vi "Render.vi"(7 "Renderer":refnum<class "Renderer.lvclass">, 8 "error in (no error)":errorcluster, 9 "Position":refnum<class "Vector 2D.lvclass">, 10 "String":string, 11 "Font in":refnum<class "Sprite Font.lvclass">) -> (0 "error out":errorcluster)   [LabVIEW 2021, in "Sprite Font.lvclass"]
uses:
  Sprite Font.lvclass
  Renderer/Renderer.lvclass
  Re-use Libraries/Vector 2D/Vector 2D.lvclass
  Sprite Font.lvclass/Sprite Font.ctl
  Re-use Libraries/Vector 2D/Vector 2D.lvclass/Vector 2D.ctl
  Renderer/Renderer.lvclass/Renderer.ctl
  Texture/Texture.lvclass/Texture.ctl
  Resource Manager/Resource Manager.lvclass
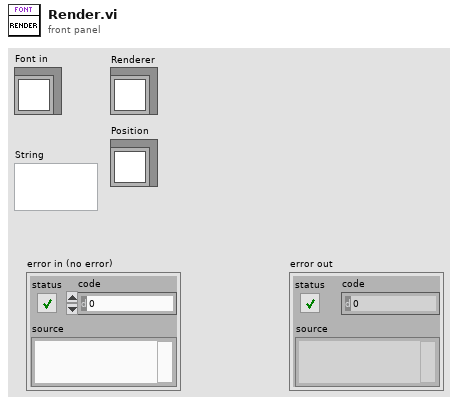
[diagram p1: front panel]
types:
  T1 = typedef "Sprite Font.lvclass/Character.ctl" = cluster{"Texture Name":string, "Size":refnum<class "Vector 2D.lvclass">}
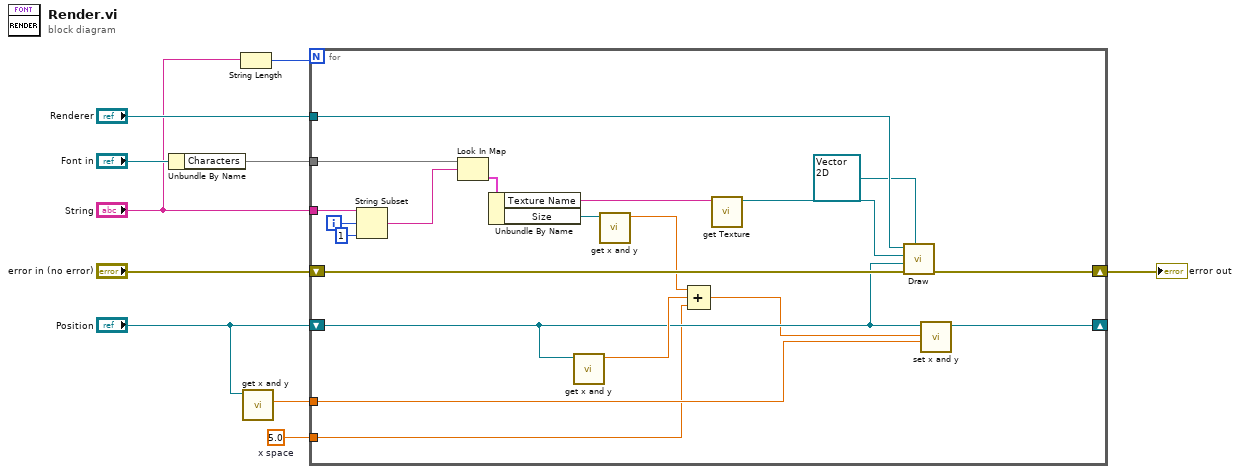
[diagram p0: block diagram]
diagram:
  w3 = sgl 5.0  # x space
  n1 = Unbundle By Name("Font in") -> ("Characters"=w6:map{string, T1})
  n2 = String Length(string="String") -> (length=w5:i32)
  n3 = call "get x and y.vi"("Vector 2D in"="Position") -> ("y"=w1:sgl)  [unwired: 9 in, 1 out]
  n4 = for {
    N: w5 -> [_]
    tunnel: "Renderer" -> [w30]
    shift-right: [w28] -> w9
    shift-left: "error in (no error)" -> [w27]
    tunnel: w6 -> [w18]
    shift-right: [w21] -> _
    shift-left: "Position" -> [w20]
    tunnel: w1 -> [w23]
    tunnel: "String" -> [w17]
    tunnel: w3 -> [w12]
    i -> [w16]
    n5 = String Subset(string=w17, offset (0)=w16, length (rest)=1 ("length (rest)")) -> (substring=w13:string)
    n6 = Look In Map(map=w18, key=w13) -> (value=w14:T1)  [unwired: 1 in, 1 out]
    n7 = Unbundle By Name(w14) -> ("Texture Name"=w25:string, "Size"=w24:refnum<class "Vector 2D.lvclass">)
    n8 = call "get x and y.vi"("Vector 2D in"=w20) -> ("x"=w22:sgl)  [unwired: 9 in, 1 out]
    n9 = call "get x and y.vi"("Vector 2D in"=w24) -> ("x"=w11:sgl)  [unwired: 9 in, 1 out]
    n10 = Compound Arithmetic op=ADD(w11, w22, w12) -> (w19:sgl)
    n11 = call "get Texture.vi"("Texture Name"=w25) -> ("Texture"=w29:refnum<class "Texture.lvclass">)  [unwired: 10 in]
    n12 = call "Draw.vi"("Rotation Center"=refnum<class "Vector 2D.lvclass"> refnum, "error in (no error)"=w27, "Destination"=w20, "Texture"=w29, "Renderer"=w30) -> ("error out"=w28:errorcluster)  [unwired: 6 in]
    n13 = call "set x and y.vi"("y"=w23, "x"=w19, "Vector 2D in"=w20) -> ("Vector 2D out"=w21:refnum<class "Vector 2D.lvclass">)  [unwired: 8 in]
  }
  "error out" <- w9
